vi "Actor Destroy Core.vi"(7 "Actor":refnum<class "Actor.lvclass">, 11 "Msging Self Actor State in":refnum<class "Msging Self Actor State.lvclass">) -> (0 "error out":errorcluster)   [LabVIEW 2021, in "LVCAM.lvlib" / "Msging Self Actor State.lvclass"]
uses:
  Msging Self Actor State.lvclass
  Actor/Actor.lvclass
  Self Actor/Self Actor.lvclass
  Msgs/Actor Destroy/Actor Destroy Msg Strategy/Actor Destroy Msg Strategy.lvclass
  C:/git/LabVIEW-Composed-Actor-Model-LVCAM/LabVIEW-Composed-Actor-Model-LVCAM/LVCAM/LVCAM/Msg Strategy/Msg Strategy.lvclass
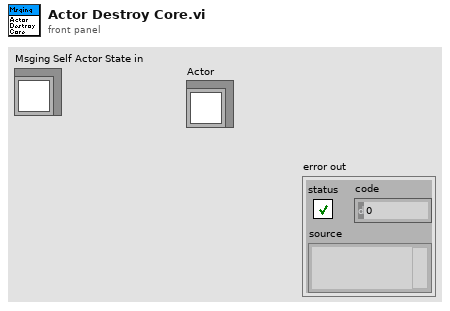
[diagram p1: front panel]
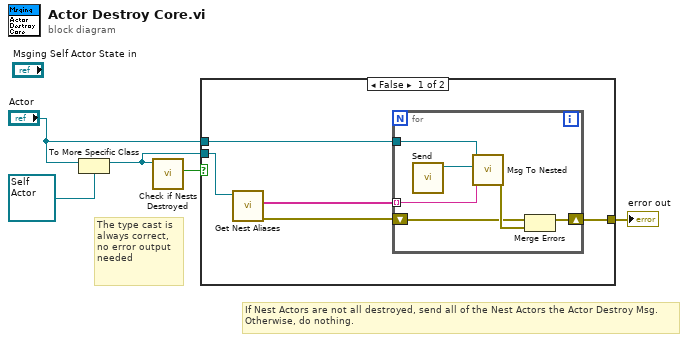
[diagram p0: block diagram]
diagram:
  # "The type cast is always correct, no error output needed"
  # "If Nest Actors are not all destroyed, send all of the Nest Actors the Actor Destroy Msg. Otherwise, do nothing."
  n1 = To More Specific Class(target class=refnum<class "Self Actor.lvclass"> refnum ("LVCAM.lvlib:Self Actor.lvclass"), reference="Actor") -> (specific class reference=w2:refnum<class "Self Actor.lvclass">)  [unwired: 1 in, 1 out]
  n2 = call "Check if Nests Destroyed.vi"("Self Actor"=w2) -> ("Nest Actors Destroyed?"=w4:bool)  [unwired: 10 in]
  n3 = case shown="False" w4 {
    tunnel: [w10 _] -> w5
    tunnel: "Actor" -> [w7 _]
    tunnel: w2 -> [w6 _]
    frame False {
      n4 = call "Get Nest Aliases.vi"("Self Actor"=w6) -> ("error out"=w8:errorcluster, "Nest Msg Q Aliases"=w9:string[])  [unwired: 9 in]
      n5 = for {
        tunnel: w9 -> [w13] mode=indexing
        shift-right: [w16] -> w10
        shift-left: w8 -> [w11]
        tunnel: w7 -> [w15]
        n6 = call "Send.vi"() -> ("Actor Destroy Msg Strategy out"=w14:refnum<class "Actor Destroy Msg Strategy.lvclass">)  [unwired: 11 in]
        n7 = call-dynamic "Msg To Nested.vi"("Alias"=w13, "Msg"=w14, "Actor in"=w15) -> ("error out"=w12:errorcluster)  [unwired: 8 in]
        n8 = Merge Errors(w11, w12) -> (w16:errorcluster)
      }
    }
    frame True {
      # "there exist no Nest Actors to be destroyed, do nothing"
    }
  }
  "error out" <- w5
